vi "Update Loaded Plugins by Reference.vi"(8 "error in (no error)":errorcluster, 10 "Plugin Summary Info":T1[](array[typedef]), 11 "Loaded Plugins ref in":refnum<vi>) -> (0 "error out":errorcluster, 3 "Loaded Plugins ref out":refnum<vi>)   [LabVIEW 2021, in "CIF_UI.lvclass"]
uses:
  CIF_UI.lvclass
  Typedef/Plugin Summary.ctl
  Typedef/Version.ctl
  CIF_UI.lvclass/CIF_UI.ctl
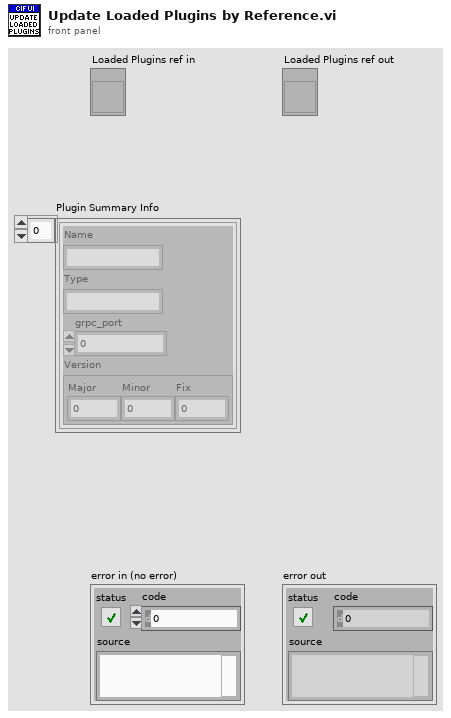
[diagram p1: front panel]
types:
  T1 = typedef "CIF_UI.lvclass/Plugin Summary.ctl" = cluster{"Name":string, "Type":string, "grpc_port":i32, "Version":T2}
  T2 = typedef "CIF_UI.lvclass/Version.ctl" = cluster{"Major":i32, "Minor":i32, "Fix":i32}
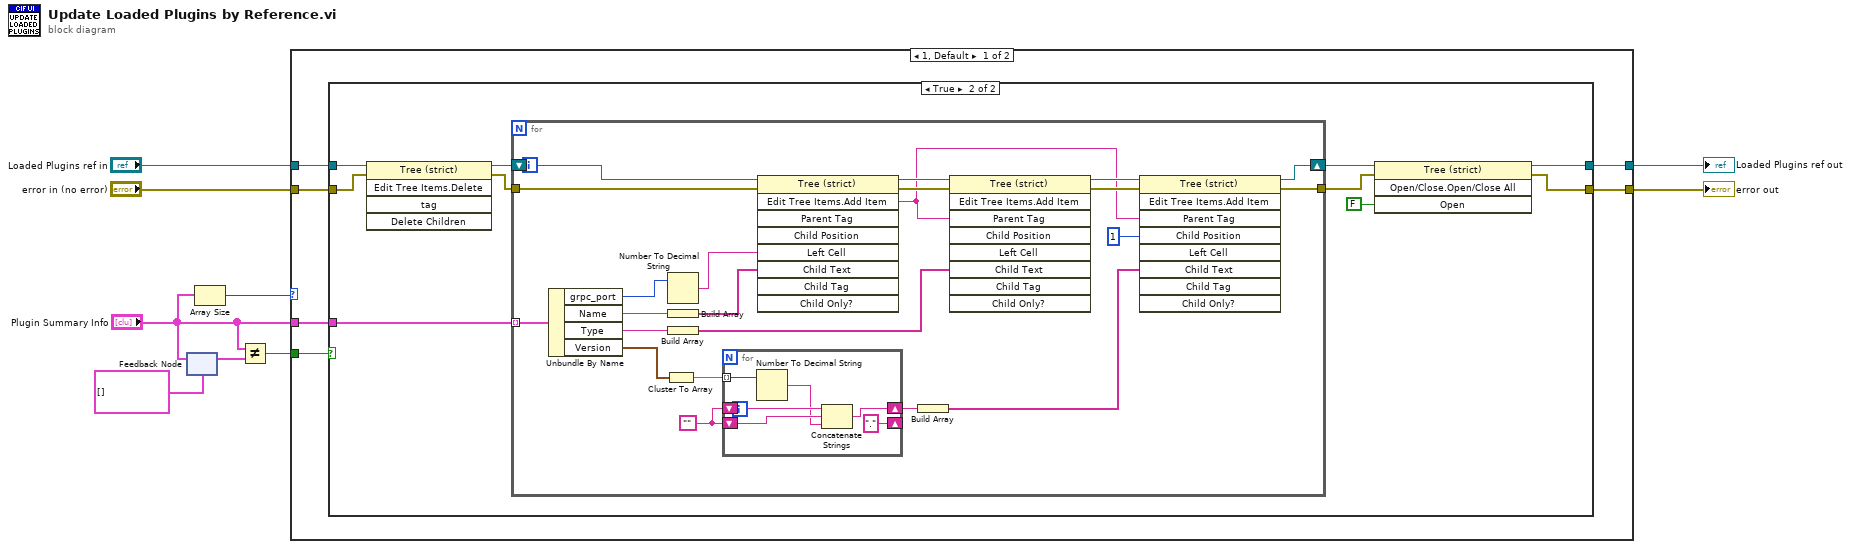
[diagram p0: block diagram]
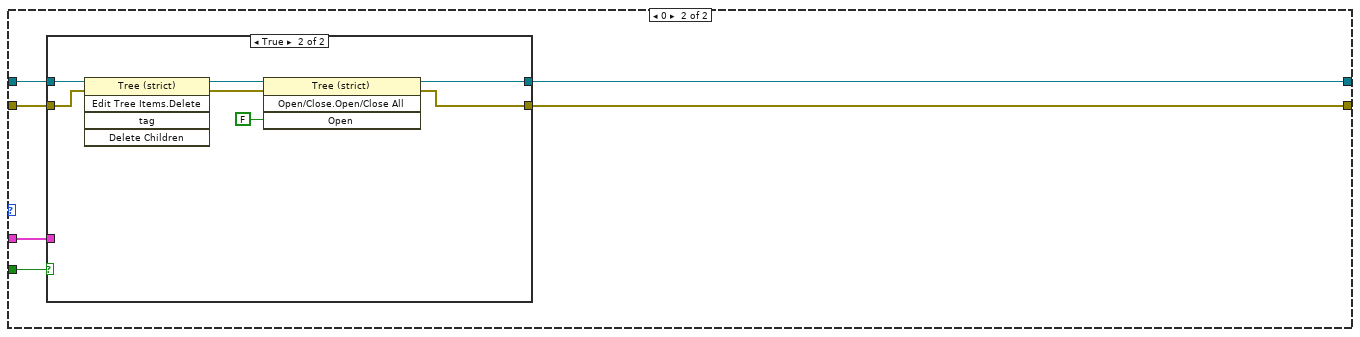
[diagram p3: hidden frame]
diagram:
  n1 = feedback #1(T1[] [] ("Sorted Plugin Info")) -> (w3:T1[])
  n2 = feedback-in #1("Plugin Summary Info") -> ()
  n3 = Array Size(array="Plugin Summary Info") -> (size(s)=w1:i32)
  n4 = Not Equal?(x="Plugin Summary Info", y=w3) -> (x != y?=w2:bool)
  n5 = case shown="1, Default" w1 {
    tunnel: "error in (no error)" -> [w15 w61]
    tunnel: [w14 w60] -> w8
    tunnel: [w13 w59] -> w7
    tunnel: "Loaded Plugins ref in" -> [w12 w58]
    tunnel: w2 -> [w11 w57]
    tunnel: "Plugin Summary Info" -> [w10 w56]
    frame 1, Default {
      n6 = case shown="True" w11 {
        tunnel: w15 -> [w16 w22]
        tunnel: [w16 w21] -> w14
        tunnel: [w17 w20] -> w13
        tunnel: w12 -> [w17 w19]
        tunnel: w10 -> [_ w18]
        frame False {
        }
        frame True {
          n7 = invoke class="Tree (strict)" method="Edit Tree Items.Delete"(reference=w19, error in=w22) -> (reference out=w26:refnum<vi>, error out=w27:errorcluster)  [unwired: 3 in, 3 out]
          n8 = for {
            tunnel: w27 -> [w32]
            tunnel: [w49] -> w24
            shift-right: [w46] -> w25
            shift-left: w26 -> [w33]
            tunnel: w18 -> [w34] mode=indexing
            w47 = ""
            n9 = Unbundle By Name(w34) -> ("grpc_port"=w35:i32, "Name"=w28:string, "Type"=w39:string, "Version"=w36:T2)
            n10 = Cluster To Array(cluster=w36) -> (array=w48:i32[])
            n11 = Number To Decimal String(number=w35) -> (decimal integer string=w40:string)  [unwired: 1 in]
            n12 = Build Array(w28) -> (w29:string[])
            n13 = Build Array(w39) -> (w31:string[])
            n14 = for {
              tunnel: w48 -> [w50] mode=indexing
              shift-right: ["."] -> _
              shift-left: w47 -> [w54]
              shift-right: [w52] -> w38
              shift-left: w47 -> [w55]
              n15 = Number To Decimal String(number=w50) -> (decimal integer string=w53:string)  [unwired: 1 in]
              n16 = Concatenate Strings(w55, w54, w53) -> (w52:string)
            }
            n17 = invoke class="Tree (strict)" method="Edit Tree Items.Add Item"(reference=w33, error in=w32, "Left Cell"=w40, "Child Text"=w29) -> (reference out=w45:refnum<vi>, error out=w44:errorcluster, "Edit Tree Items:Add Item"=w30:string)  [unwired: 5 in, 6 out]
            n18 = Build Array(w38) -> (w37:string[])
            n19 = invoke class="Tree (strict)" method="Edit Tree Items.Add Item"(reference=w45, error in=w44, "Parent Tag"=w30, "Child Text"=w31) -> (reference out=w43:refnum<vi>, error out=w42:errorcluster)  [unwired: 5 in, 7 out]
            n20 = invoke class="Tree (strict)" method="Edit Tree Items.Add Item"(reference=w43, error in=w42, "Parent Tag"=w30, "Child Position"=1, "Child Text"=w37) -> (reference out=w46:refnum<vi>, error out=w49:errorcluster)  [unwired: 4 in, 7 out]
          }
          n21 = invoke class="Tree (strict)" method="Open/Close.Open/Close All"(reference=w25, error in=w24, "Open"=FALSE ("Open?")) -> (reference out=w20:refnum<vi>, error out=w21:errorcluster)  [unwired: 1 in, 2 out]
        }
      }
    }
    frame 0 {
      n22 = case shown="True" w57 {
        tunnel: w61 -> [w62 w69]
        tunnel: [w62 w68] -> w60
        tunnel: [w63 w67] -> w59
        tunnel: w58 -> [w63 w66]
        tunnel: w56 -> [_ _]
        frame False {
        }
        frame True {
          n23 = invoke class="Tree (strict)" method="Edit Tree Items.Delete"(reference=w66, error in=w69) -> (reference out=w65:refnum<vi>, error out=w64:errorcluster)  [unwired: 3 in, 3 out]
          n24 = invoke class="Tree (strict)" method="Open/Close.Open/Close All"(reference=w65, error in=w64, "Open"=FALSE ("Open?")) -> (reference out=w67:refnum<vi>, error out=w68:errorcluster)  [unwired: 1 in, 2 out]
        }
      }
    }
  }
  "Loaded Plugins ref out" <- w7
  "error out" <- w8
